vi "cell_temp_stddev.vi"(1 "Current cell temp":dbl, 2 "Titration State":string) -> (0 "Cell Temp Std Dev":dbl)   [LabVIEW 2010]
uses:
  <vilib>/Analysis/NI_AALBase.lvlib
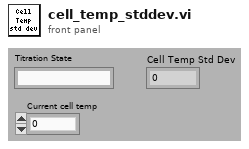
[diagram p1: front panel]
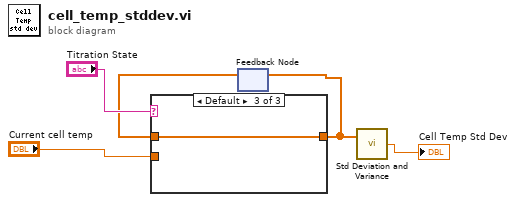
[diagram p0: block diagram]
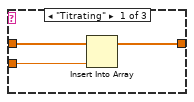
[diagram p2: hidden frame]
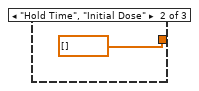
[diagram p3: hidden frame]
diagram:
  n1 = feedback #1() -> (w2:dbl[])  [unwired: 1 in]
  n2 = case shown="Default" "Titration State" {
    tunnel: "Current cell temp" -> [w8 _ _]
    tunnel: [w7 dbl[] [] w10] -> w1
    tunnel: w2 -> [w6 _ w10]
    frame "Titrating" {
      n3 = Insert Into Array(array=w6, new element=w8) -> (w7:dbl[])  [unwired: 1 in]
    }
    frame "Hold Time", "Initial Dose" {
    }
    frame Default {
    }
  }
  n4 = feedback-in #1(w1) -> ()
  n5 = call <vilib>:"Std Deviation and Variance.vi"("X"=w1) -> ("standard deviation"=→"Cell Temp Std Dev":dbl)  [unwired: 1 in, 2 out]
